vi "ToSlide.vi"(8 "error in":errorcluster, 11 "Generic":refnum<class "Generic.lvclass">) -> (0 "error out":errorcluster, 3 "Slide out":refnum<class "Slide.lvclass">)   [LabVIEW 2014, in "Slide.lvclass"]
uses:
  Slide.lvclass
  Generic/Generic.lvclass
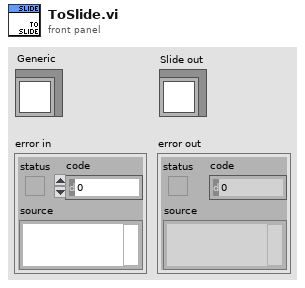
[diagram p1: front panel]
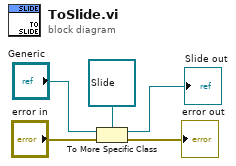
[diagram p0: block diagram]
diagram:
  n1 = To More Specific Class(target class=refnum<class "Slide.lvclass"> refnum ("Knob in"), reference="Generic", error in="error in") -> (specific class reference=→"Slide out":refnum<class "Slide.lvclass">, error out=→"error out":errorcluster)
